vi "Configure Setpoint.vi"(0 "VISA resource name":refnum<visa-resource-name>, 1 "Unit Address (1)":u8=1 min=1 max=254, 5 "Setpoint (0: Setpoint 1)":u8(ring) items=["Setpoint 1", "Setpoint 2", "Remote Setpoint", "Target Setpoint"], 9 "Setpoint Value (0)":i16, 11 "error in (no error)":errorcluster) -> (4 "VISA resource name out":refnum<visa-resource-name>, 15 "error out":errorcluster)   [LabVIEW 2010, in "Eurotherm 32xx Series.lvlib"]
doc: "This VI sets setpoint value. \n\nCaution – DO NOT WRITE continuously changing values to Setpoint 1, Setpoint 2 or Target Setpoint. The memory technology used in this product has a limited (100,000) number of write cycles. If ramped setpoints are required, consider using the internal ramp rate function or the remote comms setpoint (Modbus address 26 ) in preference.\n\nRm.SP\nRemote (comms) setpoint. If selected using the remote setpoint selection (address 276, may also be controlled using the instrument HMI or a digital input) then this is used as a setpoint providing a value has been received within a window of about 5 seconds. If no value is received then the controller falls back to the currently selected setpoint (SP 1 or SP 2) with an error indication. The Remote Setpoint may have a local trim (SP Trim, address 27) added to it to compensate for variations in temperature in a particular zone. This parameter is not saved when the instrument is switched off. It may be written to continuously over communications without risk of damage to the instrument non-volatile memory."
uses:
  <instrlib>/Eurotherm 32xx Series/Eurotherm 32xx Series.lvlib
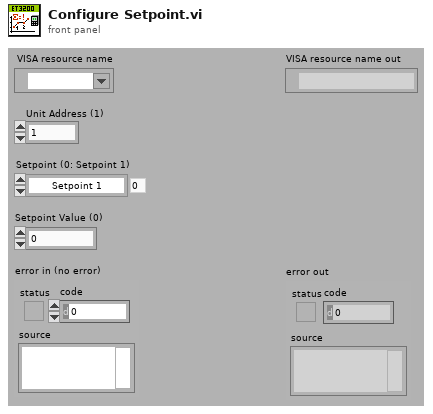
[diagram p1: front panel]
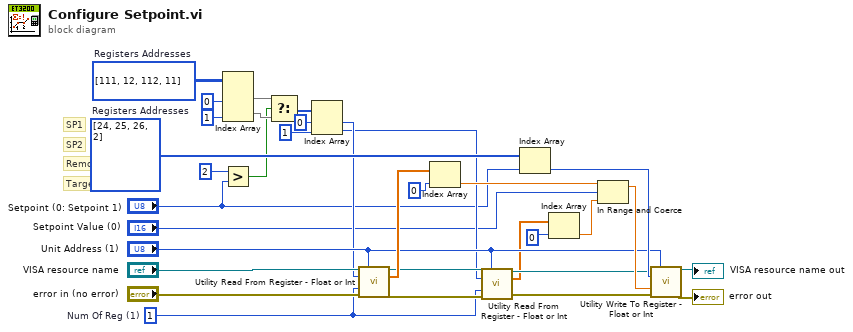
[diagram p0: block diagram]
diagram:
  w23 = u16[][] [[111, 12], [112, 11]]  # Registers Addresses
  w8 = u16 1  # Num Of Reg (1)
  w26 = u16[] [24, 25, 26, 2]  # Registers Addresses
  # "TargetSP"
  # "RemoteSP"
  # "SP2"
  # "SP1"
  n1 = Index Array(array=w23, index (col) #1=0 ("disabled index (col)"), index (col) #2=1 ("index (col)")) -> (element #1=w20:u16[], element #2=w19:u16[])  [unwired: 2 in]
  n2 = Greater?(x=u8 2, y="Setpoint (0: Setpoint 1)") -> (0:w1:bool)
  n3 = Select(t=w20, s=w1, f=w19) -> (s? t:f=w13:u16[])
  n4 = Index Array(array=w13, index #1=0 ("index"), index #2=1 ("index")) -> (element #1=w10:u16, element #2=w9:u16)
  n5 = call <instrlib>:"Utility Read From Register - Float or Int.vi"("VISA resource name"="VISA resource name", "Unit Address (1)"="Unit Address (1)", "Register Address (0)"=w10, "Num Of Reg (1)"=w8, "error in (no error)"="error in (no error)") -> ("VISA resource name out"=w18:refnum<visa-resource-name>, "Data"=w31:sgl[], "error out"=w15:errorcluster)  [unwired: 8 in]
  n6 = Index Array(array=w31, index=0) -> (element=w29:sgl)
  n7 = call <instrlib>:"Utility Read From Register - Float or Int.vi"("VISA resource name"=w18, "Unit Address (1)"="Unit Address (1)", "Register Address (0)"=w9, "Num Of Reg (1)"=w8, "error in (no error)"=w15) -> ("VISA resource name out"=w17:refnum<visa-resource-name>, "Data"=w6:sgl[], "error out"=w16:errorcluster)  [unwired: 8 in]
  n8 = Index Array(array=w26, index="Setpoint (0: Setpoint 1)") -> (element=w25:u16)
  n9 = Index Array(array=w6, index=0) -> (element=w5:sgl)
  n10 = In Range and Coerce(upper limit=w29, x="Setpoint Value (0)", lower limit=w5) -> (coerced(x)=w24:sgl)  [unwired: 1 out]
  n11 = call <instrlib>:"Utility Write To Register - Float or Int.vi"("VISA resource name"=w17, "Unit Address (1)"="Unit Address (1)", "Register Address (0)"=w25, "Data (0)"=w24, "error in (no error)"=w16) -> ("VISA resource name out"=→"VISA resource name out":refnum<visa-resource-name>, "error out"=→"error out":errorcluster)  [unwired: 9 in]
